vi "Create Custom Char.vi"(8 "error in (no error)":errorcluster, 9 "Char":T1=[[FALSE, FALSE, FALSE, FALSE, FALSE], [FALSE, FALSE, FALSE, FALSE, FALSE], [FALSE, FALSE, FALSE, FALSE, FALSE], [FALSE, FALSE, FALSE, FALSE, FALSE], [FALSE, FALSE, FALSE, FALSE, FALSE], [FALSE, FALSE, FALSE, FALSE, FALSE], [FALSE, FALSE, FALSE, FALSE, FALSE], [FALSE, FALSE, FALSE, FALSE, FALSE]], 10 "Session In":refnum<class "Session.lvclass">, 11 "Character LCD in":refnum<class "Char LCD I.lvclass">) -> (0 "error out":errorcluster, 2 "Session Out":refnum<class "Session.lvclass">, 3 "Character LCD out":refnum<class "Char LCD I.lvclass">)   [LabVIEW 2020, in "CTI-Device.lvlib" / "Char LCD I.lvclass"]
uses:
  Char LCD I.lvclass
  Custom Char.ctl
  CTI/Session/Session.lvclass
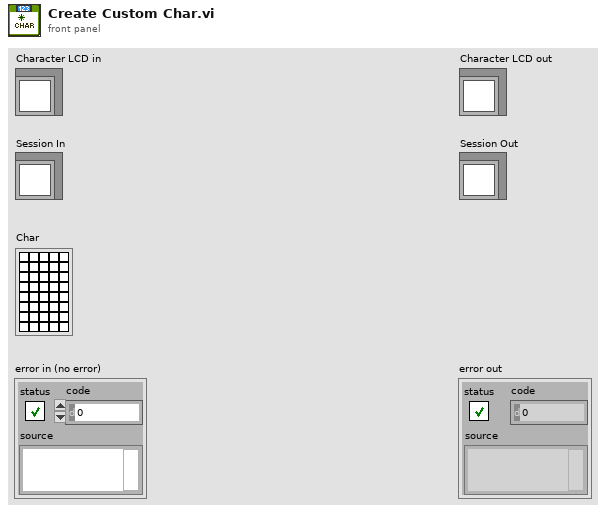
[diagram p1: front panel]
types:
  T1 = typedef "CTI-Device.lvlib/Char LCD I.lvclass/Custom Char.ctl" = bool[][]
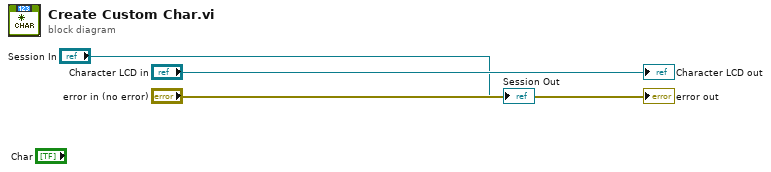
[diagram p0: block diagram]
diagram:
  "error out" <- "error in (no error)"
  "Character LCD out" <- "Character LCD in"
  "Session Out" <- "Session In"
